vi "Max RPM Value.vi"(8 "error in (no error)":errorcluster, 11 "Controller in":T1) -> (0 "error out":errorcluster, 2 "MXRPM":dbl format="%#_13g", 3 "Controller out":T1, 4 "Receive Answer":string, 5 "Sent Command":string)   [LabVIEW 2017, in "Roboteq Controller KBL1xxx.lvlib"]
uses:
  <instrlib>/Roboteq Controller KBL1xxx/Roboteq Controller KBL1xxx.lvlib
  <instrlib>/Roboteq Controller KBL1xxx/Public/Controls/Controller.ctl
  <instrlib>/Roboteq Controller KBL1xxx/Private/Support/Command Create (0 parameters).vi
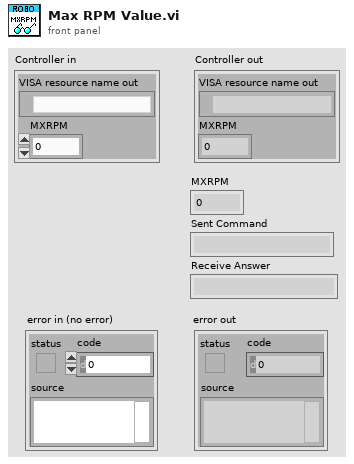
[diagram p1: front panel]
types:
  T1 = typedef "Roboteq Controller KBL1xxx.lvlib/Controller.ctl" = cluster{"VISA resource name out":refnum<visa-resource-name>, "MXRPM":u16}
  T2 = enum16{"Runtime", "Configuration", "Maintenance"}
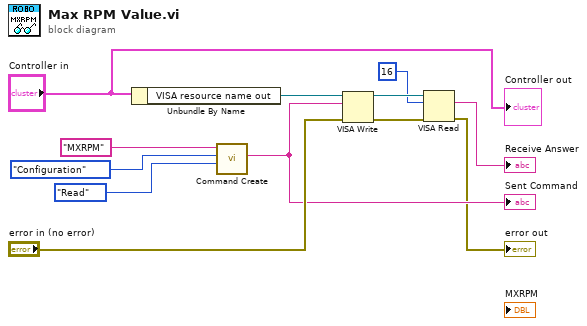
[diagram p0: block diagram]
diagram:
  n1 = Unbundle By Name("Controller in") -> ("VISA resource name out"=w9:refnum<visa-resource-name>)
  n2 = call-poly <instrlib>:"Command Create.vi"("Command Mode"=enum16{"Write", "Read"}."Read", "Command Type"=T2."Configuration", "Command Name"="MXRPM") -> ("Command"=w3:string)  [unwired: 8 in]
  "Sent Command" <- w3
  n3 = VISA Write(VISA resource name=w9, write buffer=w3, error in (no error)="error in (no error)") -> (VISA resource name out=w7:refnum<visa-resource-name>, error out=w6:errorcluster)  [unwired: 1 out]
  n4 = VISA Read(VISA resource name=w7, byte count=u32 16, error in (no error)=w6) -> (read buffer=→"Receive Answer":string, error out=→"error out":errorcluster)  [unwired: 2 out]
  "Controller out" <- "Controller in"
